vi "lib Quick Message Log.vi"(8 "error in (no error)":errorcluster, 10 "Clear":bool, 11 "Message":string) -> (0 "error out":errorcluster, 3 "Log":string)   [LabVIEW 2024]
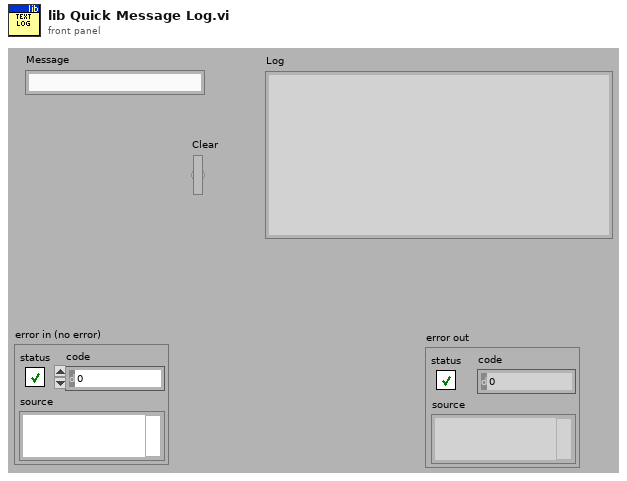
[diagram p1: front panel]
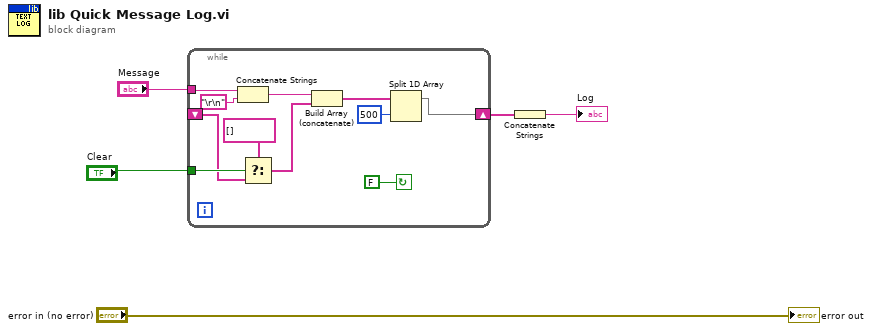
[diagram p0: block diagram]
diagram:
  n1 = while {
    shift-right: [w14] -> w2
    shift-left: _ -> [w12]
    tunnel: "Message" -> [w9]
    tunnel: "Clear" -> [w13]
    stop <- FALSE continue-if-true
    n2 = Concatenate Strings(w9, "\r\n") -> (w8:string)
    n3 = Select(t=string[] [], s=w13, f=w12) -> (s? t:f=w11:string[])
    n4 = Build Array (concatenate)(w8, w11) -> (w16:string[])
    n5 = Split 1D Array(array=w16, index=500) -> (first subarray=w14:string[])  [unwired: 1 out]
  }
  n6 = Concatenate Strings(w2) -> (→"Log":string)
  "error out" <- "error in (no error)"
